vi "8-1 컴퓨터ProcessID (DLL).vi"() -> ()   [LabVIEW 2014]
uses:
  Windows/System32/kernel32.dll
panel:
  out "ComputerName":string
  out "반환 타입":i32
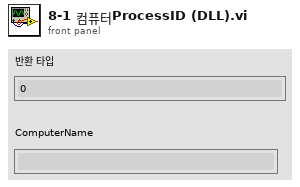
[diagram p1: front panel]
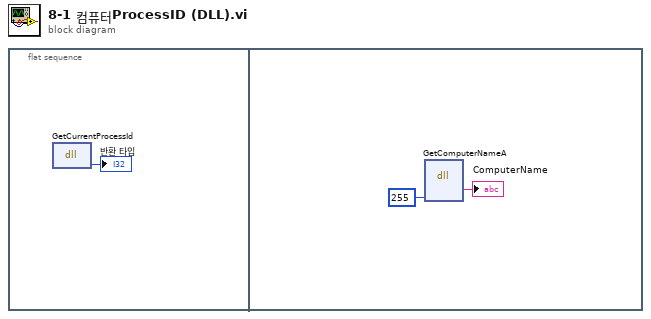
[diagram p0: block diagram]
diagram:
  n1 = flat-sequence {
    frame #0 {
      n2 = dll-call lib="C:/Windows/System32/kernel32.dll" fn="GetCurrentProcessId"() -> ("반환 타입"=→"반환 타입":i32)  [unwired: 3 in, 2 out]
    }
    frame #1 {
      n3 = dll-call lib="C:/Windows/System32/kernel32.dll" fn="GetComputerNameA"("lenth"=u32 255) -> ("ComputerName"=→"ComputerName":string)  [unwired: 6 in, 2 out]
    }
  }
